vi "To AStar Map.vi"(1 "empty value":dbl, 2 "Wall value":dbl, 3 "Obstacles":i32[][](array[numeric])) -> (0 "a star map":dbl[][](array[numeric]))   [LabVIEW 2015]
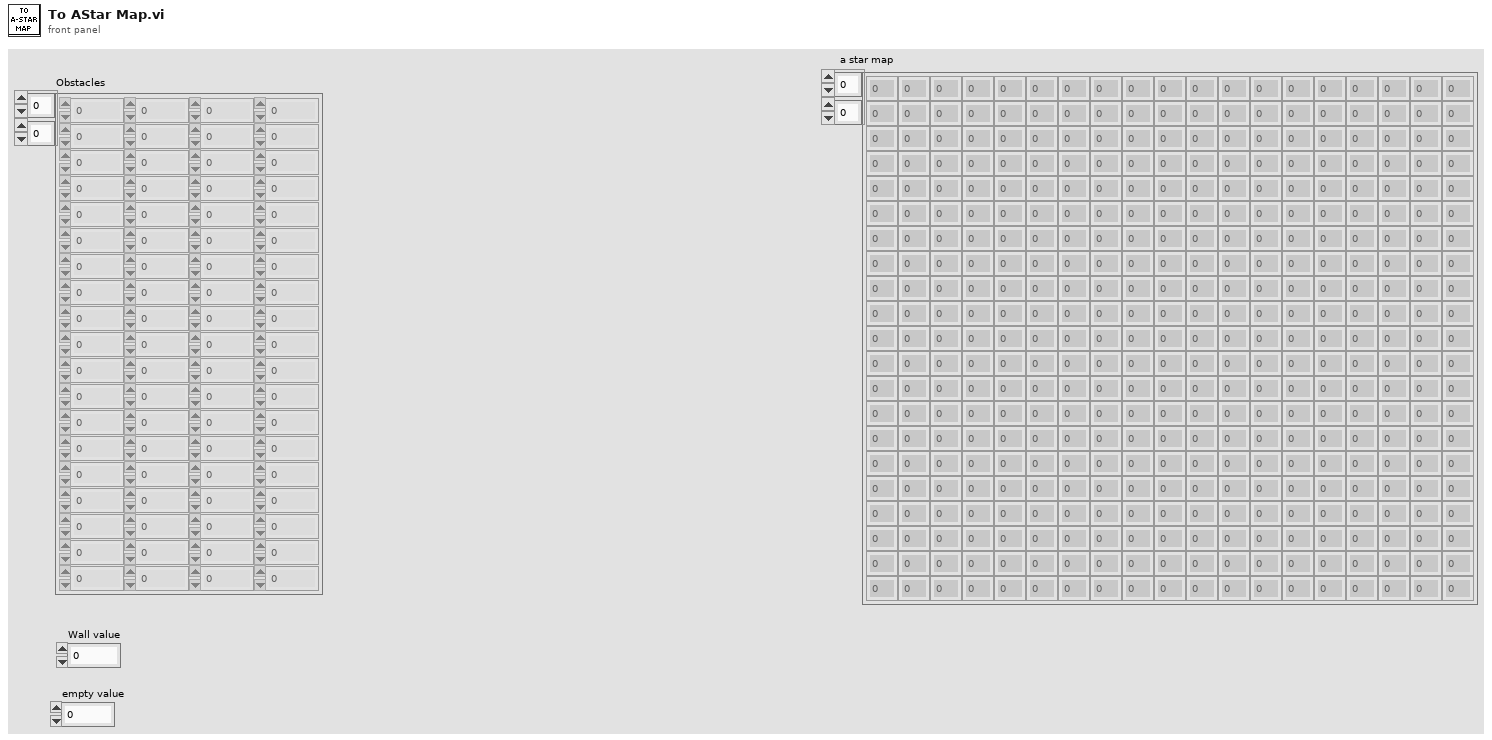
[diagram p1: front panel]
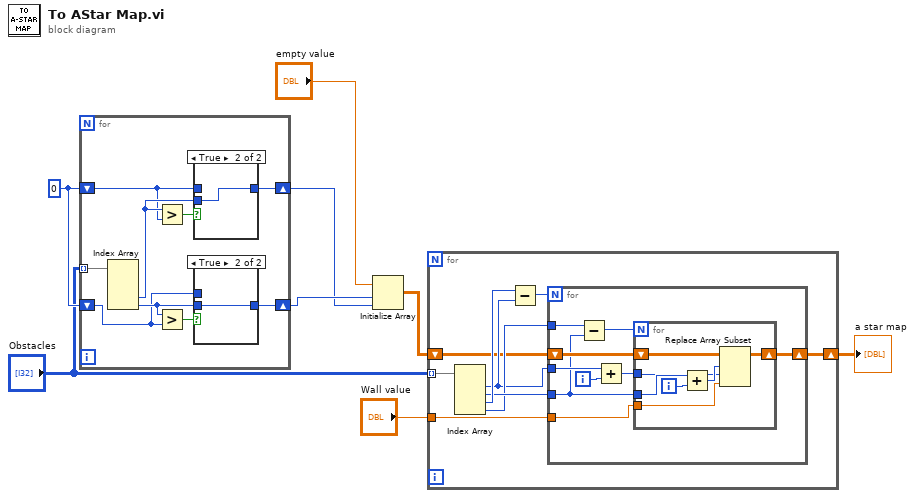
[diagram p0: block diagram]
diagram:
  w8 = 0
  n1 = for {
    tunnel: "Obstacles" -> [w17] mode=indexing
    shift-right: [w15] -> w1
    shift-left: w8 -> [w13]
    shift-right: [w11] -> w2
    shift-left: w8 -> [w9]
    n2 = Index Array(array=w17) -> (element #3=w14:i32, element #4=w10:i32)  [unwired: 4 in, 2 out]
    n3 = Greater?(x=w14, y=w13) -> (0:w16:bool)
    n4 = Greater?(x=w10, y=w9) -> (0:w12:bool)
    n5 = case shown="True" w16 {
      tunnel: [w20 w21] -> w15
      tunnel: w14 -> [_ w21]
      tunnel: w13 -> [w20 _]
      frame False {
      }
      frame True {
      }
    }
    n6 = case shown="True" w12 {
      tunnel: [w18 w19] -> w11
      tunnel: w10 -> [_ w19]
      tunnel: w9 -> [w18 _]
      frame False {
      }
      frame True {
      }
    }
  }
  n7 = Initialize Array("empty value", w2, w1) -> (w3:dbl[][])
  n8 = for {
    tunnel: "Obstacles" -> [w30] mode=indexing
    tunnel: "Wall value" -> [w24]
    shift-right: [w23] -> w4
    shift-left: w3 -> [w22]
    n9 = Index Array(array=w30) -> (element #1=w25:i32, element #2=w27:i32, element #3=w29:i32, element #4=w26:i32)  [unwired: 4 in]
    n10 = Subtract(x=w29, y=w25) -> (x-y=w28:i32)
    n11 = for {
      N: w28 -> [_]
      tunnel: w27 -> [w33]
      tunnel: w26 -> [w37]
      tunnel: w25 -> [w35]
      tunnel: w24 -> [w32]
      shift-right: [w31] -> w23
      shift-left: w22 -> [w38]
      i -> [w36]
      n12 = Subtract(x=w37, y=w33) -> (x-y=w39:i32)
      n13 = Add(x=w35, y=w36) -> (x+y=w34:i32)
      n14 = for {
        N: w39 -> [_]
        tunnel: w34 -> [w40]
        tunnel: w33 -> [w44]
        tunnel: w32 -> [w43]
        shift-right: [w42] -> w31
        shift-left: w38 -> [w46]
        i -> [w45]
        n15 = Add(x=w44, y=w45) -> (x+y=w41:i32)
        n16 = Replace Array Subset(array=w46, new element=w43, index (row)=w41, index (col)=w40) -> (w42:dbl[][])
      }
    }
  }
  "a star map" <- w4
